vi "ASK_16_MT.vi"() -> ()   [LabVIEW 2015]
uses:
  C:/Users/student/Desktop/Control 2.ctl
  <vilib>/addons/Modulation/Digital/General/MT Generate Bits (Galois, PN Order).vi
  <vilib>/addons/Modulation/Digital/Support/Common/Validators/mod_Generate Bits Validate.vi
  <vilib>/addons/Modulation/Analog/support/mod_Set Error Source.vi
  <vilib>/addons/Modulation/Digital/General/MT Generate ASK system parameters (M).vi
  <vilib>/addons/Modulation/Digital/General/subVIs/mod_Generate Bits PN Sequence.vi
  <vilib>/addons/Modulation/Digital/Support/Common/Validators/mod_Generate Filter Coefficients Validate.vi
  <vilib>/addons/Modulation/Digital/General/subVIs/mod_Generate Filter Coefficients.vi
  <vilib>/addons/Modulation/Analog/MT Upconvert Baseband (Real).vi
  <instrlib>/niUSRP/niUSRP Write Tx Data (CDB WDT).vi
  <vilib>/addons/Modulation/niDMT.lvlib
  <vilib>/addons/Modulation/niAMT.lvlib
panel:
  out "Waveform Graph":dbl[](graph)
  out "error out":errorcluster
  out "Modulated":T1
  in  "y":bool
  in  "symbol rate (Hz)":dbl=1.0 format="%.2f"
  in  "pulse shaping filter (none)":T2(ring)
  in  "M-ASK":i32=2
  out "coerced gain":dbl format="%#_6f"
  out "coerced carrier frequency":dbl=100000.0 format="%#_6p"
  out "coerced IQ rate":dbl=100000.0 format="%#_6p"
  in  "active antenna":string
  in  "gain":dbl format="%#_6f"
  in  "carrier frequency":dbl=100000.0 format="%#_6p"
  in  "IQ rate":dbl=100000.0 format="%#_6p"
  in  "device names":refnum<k15>
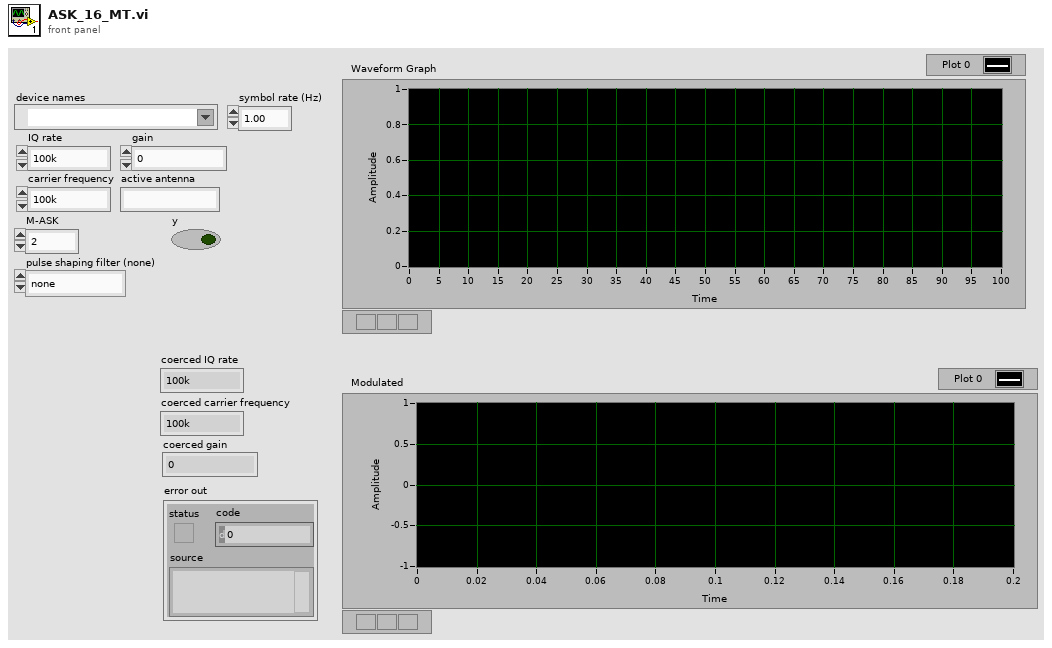
[diagram p1: front panel]
types:
  T1 = typedef "Control 2.ctl" = waveform(dbl)
  T2 = enum16{"none", "Raised Cosine", "Root Raised Cos", "Gaussian"}
  T3 = enum16{"FSK", "PSK", "QAM", "MSK", "PAM", "ASK", "CPM"}
  T4 = cluster{"samples per symbol (16)":i32, "symbol map":cdb[]}
  T5 = typedef "niAMT.lvlib/Complex Data Waveform.ctl" = cluster{"t0":dbl, "dt":dbl, "Y":cdb[]}
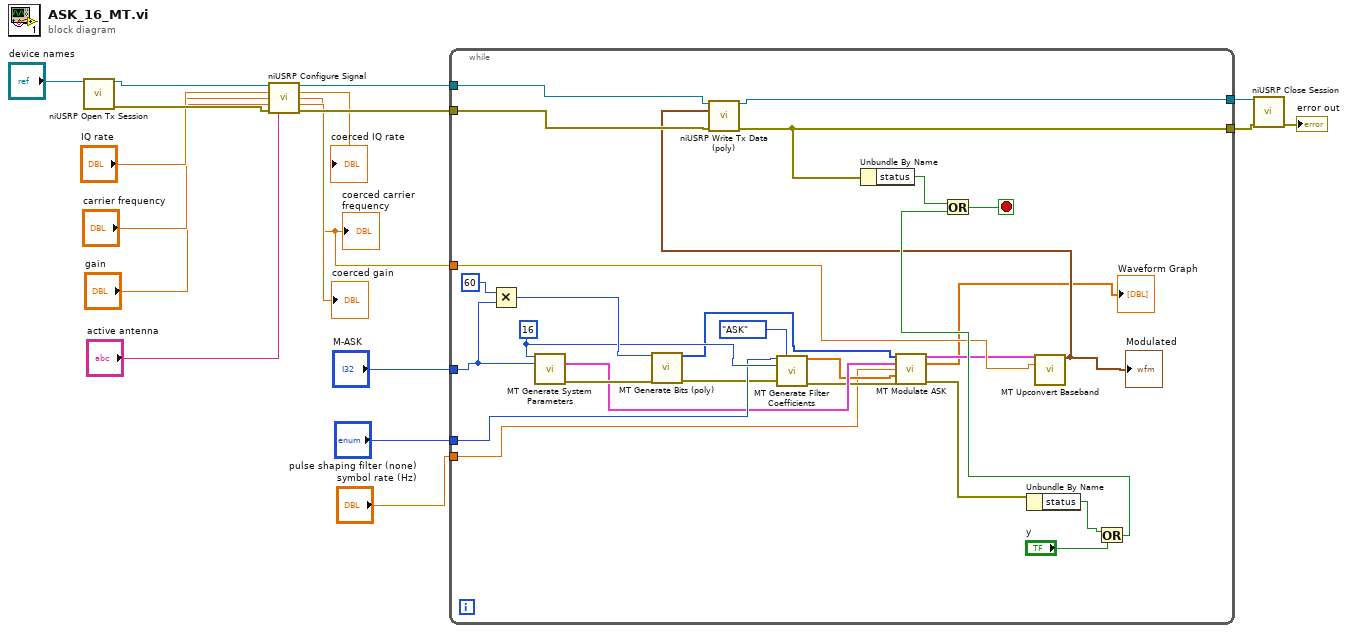
[diagram p0: block diagram]
diagram:
  n1 = call <instrlib>:"niUSRP Open Tx Session.vi"("device names"="device names") -> ("session handle out"=w14:refnum<k15>, "error out"=w18:errorcluster)  [unwired: 13 in]
  n2 = call <instrlib>:"niUSRP Configure Signal.vi"("session handle"=w14, "IQ rate"="IQ rate", "carrier frequency"="carrier frequency", "gain"="gain", "error in (no error)"=w18, "active antenna"="active antenna") -> ("session handle out"=w13:refnum<k15>, "coerced IQ rate"=→"coerced IQ rate":dbl, "coerced carrier frequency"=w2:dbl, "coerced gain"=→"coerced gain":dbl, "error out"=w17:errorcluster)  [unwired: 5 in]
  "coerced carrier frequency" <- w2
  n3 = while {
    tunnel: w17 -> [w45]
    tunnel: [w26] -> w16
    tunnel: w13 -> [w44]
    tunnel: [w43] -> w12
    tunnel: "M-ASK" -> [w41]
    tunnel: "pulse shaping filter (none)" -> [w37]
    tunnel: "symbol rate (Hz)" -> [w31]
    tunnel: w2 -> [w22]
    stop <- w23 stop-if-true
    w38 = 16 ("samples per symbol (16)")
    n4 = Multiply(x=60, y=w41) -> (x*y=w39:i32)
    n5 = call-poly <vilib>:"MT Generate System Parameters.vi"("samples per symbol (16)"=w38, "M-ASK (2)"=w41) -> ("ASK system parameters"=w34:T4, "error out"=w42:errorcluster)  [unwired: 11 in, 1 out]
    n6 = call-poly <vilib>:"MT Generate Bits (poly).vi"("total bits (128)"=w39, "error in (no error)"=w42) -> ("output bit stream"=w30:i8[], "error out"=w36:errorcluster)  [unwired: 11 in, 1 out]
    n7 = call <vilib>:"MT Generate Filter Coefficients.vi"("pulse shaping filter (none)"=w37, "modulation type"=T3."ASK", "pulse shaping samples per symbol (16)"=w38, "error in (no error)"=w36) -> ("pulse shaping filter coefficients"=w32:dbl[], "error out"=w33:errorcluster)  [unwired: 9 in, 1 out]
    n8 = call <vilib>:"MT Modulate ASK.vi"("input bit stream"=w30, "ASK system parameters"=w34, "symbol rate (Hz)"=w31, "pulse shaping filter coefficients"=w32, "error in (no error)"=w33) -> ("output complex waveform"=w21:T5, "symbols out"=→"Waveform Graph":cdb[], "error out"=w27:errorcluster)  [unwired: 8 in]
    n9 = Unbundle By Name(w27) -> ("status"=w29:bool)
    n10 = call-poly <vilib>:"MT Upconvert Baseband.vi"("baseband waveform (complex)"=w21, "carrier frequency (Hz)"=w22) -> ("passband waveform"=w20:waveform(dbl))  [unwired: 12 in, 1 out]
    "Modulated" <- w20
    n11 = call-poly <instrlib>:"niUSRP Write Tx Data (poly).vi"("session handle"=w44, "data"=w20, "error in (no error)"=w45) -> ("session handle out"=w43:refnum<k15>, "error out"=w26:errorcluster)  [unwired: 11 in]
    n12 = Unbundle By Name(w26) -> ("status"=w25:bool)
    n13 = Or(x=w29, y="y") -> (x .or. y?=w24:bool)
    n14 = Or(x=w25, y=w24) -> (x .or. y?=w23:bool)
  }
  n15 = call <instrlib>:"niUSRP Close Session.vi"("session handle"=w12, "error in (no error)"=w16) -> ("error out"=→"error out":errorcluster)  [unwired: 13 in]
